vi "Channel Selection GUI.vi"(8 "error in (no error)":errorcluster, 11 "StartNode":refnum<k24>) -> (0 "error out":errorcluster, 1 "IDs":u64[](array[numeric]), 3 "Apply":bool)   [LabVIEW 2026]
uses:
  NationalInstruments.VeriStand.SystemStorage
  NationalInstruments.VeriStand.SystemStorageUI
  WebPage Addon System Explorer.lvlib
panel:
  in  "Cancel":bool
  in  "Select":bool
  in  "TreeBrowserWF":refnum<k24>(container)
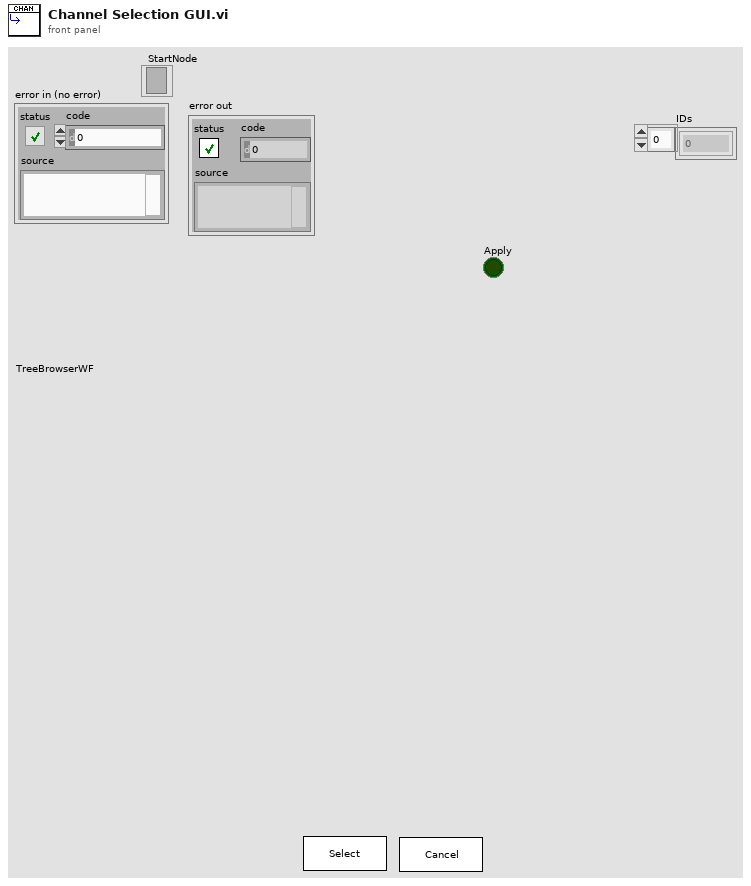
[diagram p1: front panel]
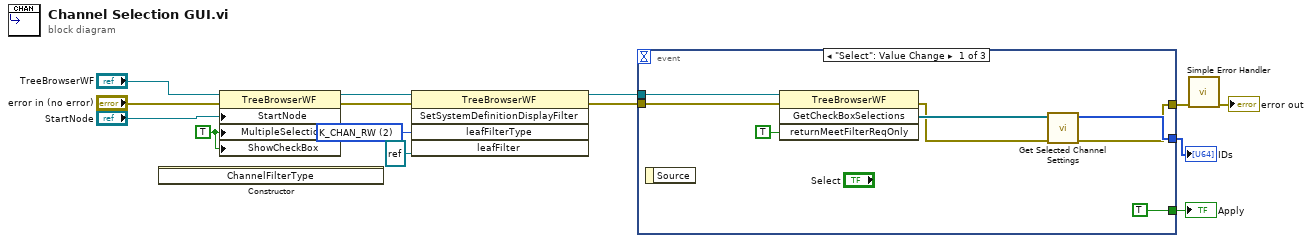
[diagram p0: block diagram]
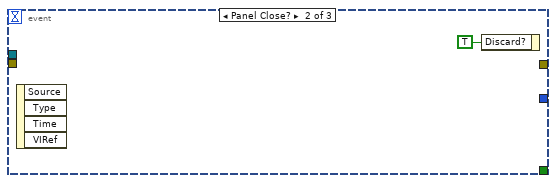
[diagram p2: hidden frame]
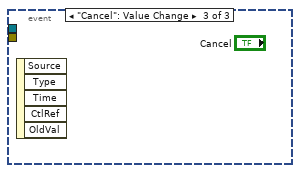
[diagram p3: hidden frame]
diagram:
  w2 = TRUE ("MultipleSelection")
  w4 = u8 2 items=["K_CHAN_R", "K_CHAN_W", "K_CHAN_RW", "K_CHAN_VOLT", "K_CHAN_FAULT", "K_ALL", "K_CUSTOM", "K_CHAN_R_VIS", "K_CHAN_W_VIS", "K_CHAN_RW_VIS", "K_CHAN_VOLT_VIS", "K_CHAN_FAULT_VIS", "K_WAVE", "K_WAVE_VIS", "K_WAVE_DBL", "K_WAVE_CDB", "K_WAVE_DBL_VIS", "K_WAVE_CDB_VIS"] ("leafFilterType")
  n1 = constructor class="TravNdMatchChannelFilter+Channe"() -> ()  [unwired: 3 in, 3 out]
  n2 = property class="TreeBrowserWF"(reference="TreeBrowserWF", error in="error in (no error)", "StartNode"="StartNode", "MultipleSelection"=w2, "ShowCheckBox"=w2) -> (reference out=w8:refnum<k24>, error out=w7:errorcluster)
  n3 = invoke class="TreeBrowserWF" method="SetSystemDefinitionDisplayFilter"(reference=w8, error in=w7, "leafFilterType"=w4, "leafFilter"=refnum<k24> refnum) -> (reference out=w6:refnum<k24>, error out=w5:errorcluster)  [unwired: 1 in, 3 out]
  n4 = event shown="[0] \"Select\": Value Change" {
    selector: _ -> [_ _ _]
    dyn-events: _ -> [_ _ _]
    timeout: _ -> [_ _ _]
    tunnel: w6 -> [w21 _ _]
    tunnel: [w20 _ _] -> w1
    tunnel: [w18 _ _] -> w14
    tunnel: w5 -> [w16 _ _]
    tunnel: [TRUE _ _] -> w9
    event "Select": Value Change {
      n5 = event-data() -> ()  [unwired: 1 in, 1 out]
      n6 = invoke class="TreeBrowserWF" method="GetCheckBoxSelections"(reference=w21, error in=w16, "returnMeetFilterReqOnly"=TRUE) -> (error out=w19:errorcluster, "GetCheckBoxSelections"=w22:refnum<k24>[])  [unwired: 1 in, 2 out]
      n7 = call "Get Selected Channel Settings.vi"("error in (no error)"=w19, "GetCheckBoxSelections"=w22) -> ("error out"=w18:errorcluster, "Array"=w20:u64[])  [unwired: 6 in, 2 out]
    }
    event Panel Close? {
      n8 = event-data() -> ()  [unwired: 1 in, 4 out]
      n9 = event-data("Discard?"=TRUE) -> ()  [unwired: 1 in, 1 out]
    }
    event "Cancel": Value Change {
      n10 = event-data() -> ()  [unwired: 1 in, 5 out]
    }
  }
  "IDs" <- w1
  "Apply" <- w9
  n11 = call <vilib>:"Simple Error Handler.vi"("error in (no error)"=w14) -> ("error out"=→"error out":errorcluster)  [unwired: 4 in, 4 out]
